vi "Add To DAQmx Task.vi"(6 "Ignore Cal? (F)":bool, 7 "Current in":refnum<class "Current.lvclass">, 8 "error in (no error)":errorcluster, 9 "Scale Name":string, 10 "Chassis Name":string, 11 "task in":refnum<k21>) -> (0 "error out":errorcluster, 2 "Phys Chan Added":string, 3 "task out":refnum<k21>)   [LabVIEW 2012, in "Measurement Channels.lvlib" / "Current.lvclass"]
uses:
  Current.lvclass
  Current.lvclass/Current.ctl
  Class Channel/Read ChanName.vi
  Class Channel/Read Alias.vi
  Class Channel/Read Scale.vi
  Class Channel/Read Offset.vi
  Class Channel/Read Unit_EU.vi
  <vilib>/DAQmx/create/scale.llb/DAQmx Create Scale (Linear).vi
  <vilib>/DAQmx/create/channels.llb/DAQmx Create Channel (AI-Current-Basic).vi
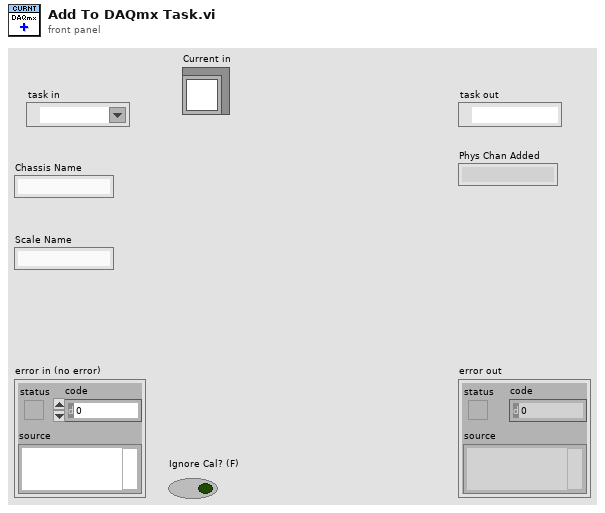
[diagram p1: front panel]
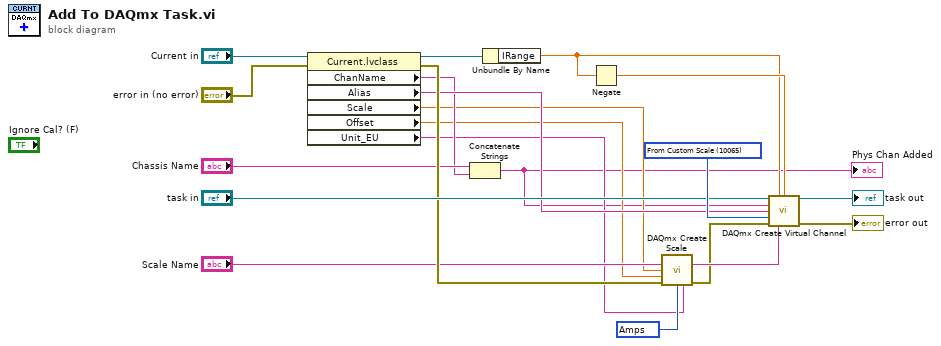
[diagram p0: block diagram]
diagram:
  w19 = 10342 items=["Volts"=10348, "Amps"=10342, "Deg F"=10144, "Deg C"=10143, "Deg R"=10145, "Kelvins"=10325, "Strain"=10299, "Ohms"=10384, "Hz"=10373, "Seconds"=10364, "Meters"=10219, "Inches"=10379, "Degrees"=10146, "Radians"=10273, "Ticks"=10304, "g"=10186, "m/s^2"=12470, "m/s"=15959, "in/s"=15960, "Pascals"=10081, "Newtons"=15875, "Pounds"=15876, "kgf"=15877, "psi"=15879, "bar"=15880, "Nm"=15881, "oz-in"=15882, "lb-in"=15883, "lb-ft"=15884, "Volts/Volt"=15896, "mVolts/Volt"=15897, "From TEDS"=12516] ("pre-scaled units")
  w18 = 10065 items=["Volts"=10348, "From Custom Scale"=10065] ("units")
  n1 = property class="Current.lvclass"(reference="Current in", error in="error in (no error)") -> (reference out=w11:refnum<class "Current.lvclass">, error out=w9:errorcluster, "ChanName"=w5:string, "Alias"=w8:string, "Scale"=w4:dbl, "Offset"=w3:dbl, "Unit_EU"=w2:string)
  n2 = Concatenate Strings("Chassis Name", w5) -> (w1:string)
  "Phys Chan Added" <- w1
  n3 = Unbundle By Name(w11) -> ("IRange"=w16:dbl)
  n4 = Negate(x=w16) -> (-x=w17:dbl)
  n5 = call-poly <vilib>:"DAQmx Create Scale.vi"("name"="Scale Name", "slope"=w4, "y-intercept"=w3, "error in"=w9, "pre-scaled units"=w19, "scaled units"=w2) -> ("scale out"=w21:tag, "error out"=w20:errorcluster)  [unwired: 8 in]
  n6 = call-poly <vilib>:"DAQmx Create Virtual Channel.vi"("task in"="task in", "maximum value"=w16, "minimum value"=w17, "physical channels"=w1, "name to assign"=w8, "units"=w18, "error in"=w20, "custom scale name"=w21) -> ("task out"=→"task out":refnum<k21>, "error out"=→"error out":errorcluster)  [unwired: 6 in]
